vi "IO参数设置.vi"(8 "布尔文本.文本":string, 9 "section (optional)":string, 10 "监测项描述":string) -> (2 "增加？":bool, 3 "簇1输出":T1)   [LabVIEW 2016, in "环境动力监测库.lvlib"]
uses:
  <vilib>/Utility/miscctls.llb/LVPointTypeDef.ctl
  <vilib>/Utility/config.llb/NI_LVConfig.lvlib
panel:
  in  "声光告警启用":bool caption="声光告警"
  in  "参数配置":bool
  in  "采集设备":enum16{"PLC", "ZLAN", "ART"}(ring)
  in  "簇1输入":T1
  in  "返回":bool
  in  "增加":bool
  in  "告警参数":enum32{"禁用告警", "闭合告警", "断开告警"}(radio)
  in  "端口":T2(ring)
  in  "监测项描述":string
  # "基本设置"
  # "如:红外XX"
  # "传感器选择"
  # "端口选择"
  # "告警方式选择"
  # "声光告警选择"
  # "参数设置"
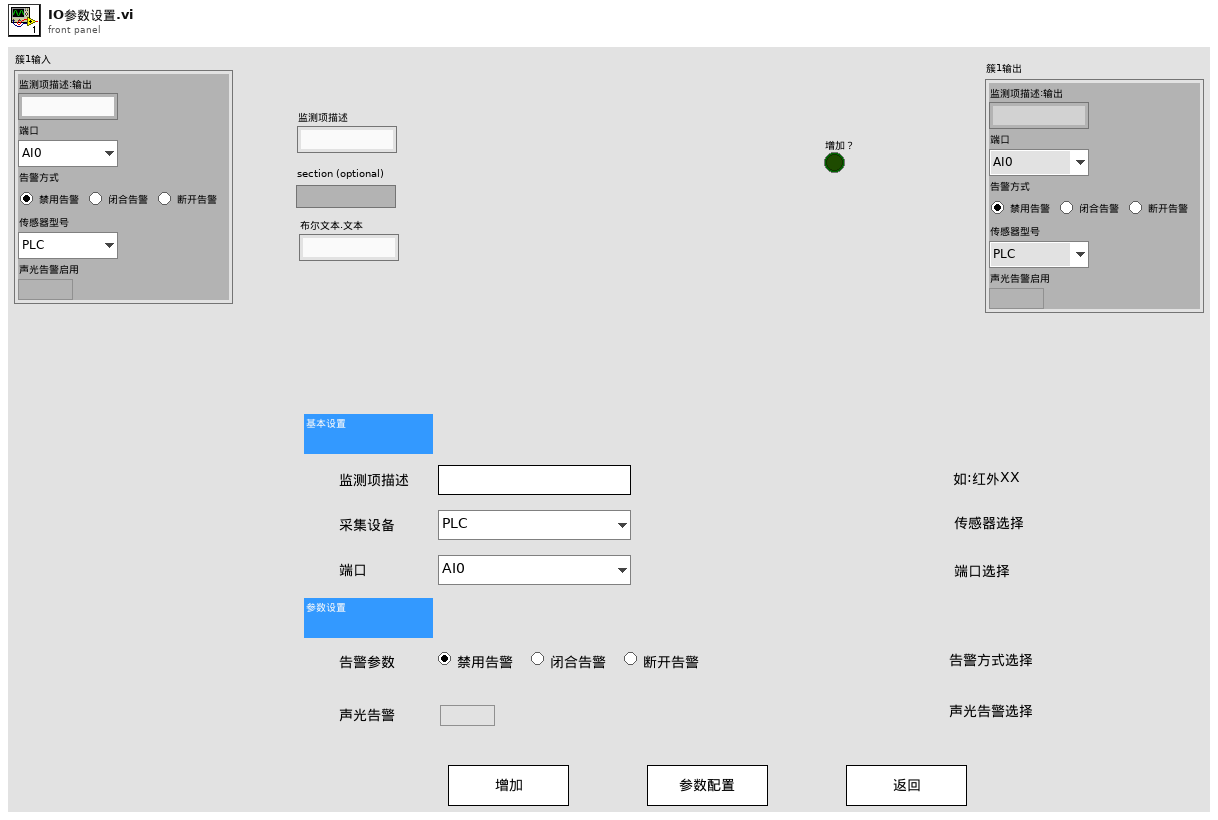
[diagram p1: front panel]
types:
  T1 = cluster{"监测项描述:输出":string, "端口":enum16{"AI0", "AI1", "AI2", "AI3", "AI4", "DI0", "DI1", "DI2", "DI3", "DI4", "DO0", "DO1", "DO2", "DO3", "DO4", "X0", "X1", "X2", "X3", "X4", "X5", "X6", "X7", "X8", "X9", "X10", "X11", "X12", "X13", "X14", "X15", "X16", "X17", "X18", "X19", "X20", "X21", "X22", "X23"}, "告警方式":enum32{"禁用告警", "闭合告警", "断开告警"}, "传感器型号":enum16{"PLC", "ZLAN", "ART"}, "声光告警启用":bool}
  T2 = enum16{"AI0", "AI1", "AI2", "AI3", "AI4", "DI0", "DI1", "DI2", "DI3", "DI4", "DO0", "DO1", "DO2", "DO3", "DO4", "X0", "X1", "X2", "X3", "X4", "X5", "X6", "X7", "X8", "X9", "X10", "X11", "X12", "X13", "X14", "X15", "X16", "X17", "X18", "X19", "X20", "X21", "X22", "X23"}
  T3 = cluster{"模板选择:":enum16{"定时简报", "无(不告警)", "通用声光告警", "通用语言告警", "通用短信告警", "通用电话告警", "通用邮件告警", "通用声光+语音+短信告警", "通用声光+短信+电话告警", "通用多方式告警", "通用全方式告警", "自动按类型", "非告警时段", "自定义"}, "预警保持时间\n(s):":i16, "重复告警时间\n(s):":i16, "告警发送方式:":cluster{"声光":bool, "语音":bool, "短信":bool, "彩信":bool, "电话":bool, "邮件":bool, "联动1":bool, "联动2":bool}, "告警时段选择:":enum16{"全时段告警", "工作日告警", "周六周日告警", "非告警时段", "自定义"}, "告警抓拍设置:":enum16{"无"}, "告警短信内容:":string, "告警电话内容:":string, "告警解除方式:":cluster{"声光":bool, "语音":bool, "短信":bool, "彩信":bool, "电话":bool, "邮件":bool, "联动1":bool, "联动2":bool}, "告警解除内容:":string, "信息接收人:":cluster{"管理员":bool, "普通用户":bool}}
  T4 = typedef "LVPointTypeDef.ctl" = cluster{"Horizontal":i16, "Vertical":i16}
  T5 = typedef "NI_LVConfig.lvlib/Config Data RefNum.ctl" = refnum<k1>
  T6 = enum8{"Enabled", "Disabled", "Disabled and Grayed Out"}
  T7 = cluster{"漏水监测配置":cluster{"监测项描述:输出":string, "端口:":enum16{"AI0", "AI1", "AI2", "AI3", "AI4", "DI0", "DI1", "DI2", "DI3", "DI4", "DO0", "DO1", "DO2", "DO3", "DO4", "X0", "X1", "X2", "X3", "X4", "X5", "X6", "X7", "X8", "X9", "X10", "X11", "X12", "X13", "X14", "X15", "X16", "X17", "X18", "X19", "X20", "X21", "X22", "X23"}, "告警参数:":enum32{"禁用告警", "闭合告警", "断开告警"}, "传感器型号:":enum16{"PLC", "ZLAN", "ART"}, "声光告警启用":bool}, "门禁开关监测配置":cluster{"监测项描述:输出":string, "端口:":enum16{"AI0", "AI1", "AI2", "AI3", "AI4", "DI0", "DI1", "DI2", "DI3", "DI4", "DO0", "DO1", "DO2", "DO3", "DO4", "X0", "X1", "X2", "X3", "X4", "X5", "X6", "X7", "X8", "X9", "X10", "X11", "X12", "X13", "X14", "X15", "X16", "X17", "X18", "X19", "X20", "X21", "X22", "X23"}, "告警参数:":enum32{"禁用告警", "闭合告警", "断开告警"}, "传感器型号:":enum16{"PLC", "ZLAN", "ART"}, "声光告警启用":bool}, "门禁开关监测配置2":cluster{"监测项描述:输出":string, "端口:":enum16{"AI0", "AI1", "AI2", "AI3", "AI4", "DI0", "DI1", "DI2", "DI3", "DI4", "DO0", "DO1", "DO2", "DO3", "DO4", "X0", "X1", "X2", "X3", "X4", "X5", "X6", "X7", "X8", "X9", "X10", "X11", "X12", "X13", "X14", "X15", "X16", "X17", "X18", "X19", "X20", "X21", "X22", "X23"}, "告警参数:":enum32{"禁用告警", "闭合告警", "断开告警"}, "传感器型号:":enum16{"PLC", "ZLAN", "ART"}, "声光告警启用":bool}, "温湿度监测配置":cluster{"监测项描述:输出":string, "端口:":enum16{"AI0", "AI1", "AI2", "AI3", "AI4", "DI0", "DI1", "DI2", "DI3", "DI4", "DO0", "DO1", "DO2", "DO3", "DO4", "X0", "X1", "X2", "X3", "X4", "X5", "X6", "X7", "X8", "X9", "X10", "X11", "X12", "X13", "X14", "X15", "X16", "X17", "X18", "X19", "X20", "X21", "X22", "X23"}, "告警参数:":enum32{"禁用告警", "闭合告警", "断开告警"}, "传感器型号:":enum16{"PLC", "ZLAN", "ART"}, "声光告警启用":bool}, "烟雾监测配置":cluster{"监测项描述:输出":string, "端口:":enum16{"AI0", "AI1", "AI2", "AI3", "AI4", "DI0", "DI1", "DI2", "DI3", "DI4", "DO0", "DO1", "DO2", "DO3", "DO4", "X0", "X1", "X2", "X3", "X4", "X5", "X6", "X7", "X8", "X9", "X10", "X11", "X12", "X13", "X14", "X15", "X16", "X17", "X18", "X19", "X20", "X21", "X22", "X23"}, "告警参数:":enum32{"禁用告警", "闭合告警", "断开告警"}, "传感器型号:":enum16{"PLC", "ZLAN", "ART"}, "声光告警启用":bool}, "冰箱监测配置":cluster{"监测项描述:输出":string, "端口:":enum16{"AI0", "AI1", "AI2", "AI3", "AI4", "DI0", "DI1", "DI2", "DI3", "DI4", "DO0", "DO1", "DO2", "DO3", "DO4", "X0", "X1", "X2", "X3", "X4", "X5", "X6", "X7", "X8", "X9", "X10", "X11", "X12", "X13", "X14", "X15", "X16", "X17", "X18", "X19", "X20", "X21", "X22", "X23"}, "告警参数:":enum32{"禁用告警", "闭合告警", "断开告警"}, "传感器型号:":enum16{"PLC", "ZLAN", "ART"}, "声光告警启用":bool}, "排气扇监测配置":cluster{"监测项描述:输出":string, "端口:":enum16{"AI0", "AI1", "AI2", "AI3", "AI4", "DI0", "DI1", "DI2", "DI3", "DI4", "DO0", "DO1", "DO2", "DO3", "DO4", "X0", "X1", "X2", "X3", "X4", "X5", "X6", "X7", "X8", "X9", "X10", "X11", "X12", "X13", "X14", "X15", "X16", "X17", "X18", "X19", "X20", "X21", "X22", "X23"}, "告警参数:":enum32{"禁用告警", "闭合告警", "断开告警"}, "传感器型号:":enum16{"PLC", "ZLAN", "ART"}, "声光告警启用":bool}, "红外入侵监测配置":cluster{"监测项描述:输出":string, "端口:":enum16{"AI0", "AI1", "AI2", "AI3", "AI4", "DI0", "DI1", "DI2", "DI3", "DI4", "DO0", "DO1", "DO2", "DO3", "DO4", "X0", "X1", "X2", "X3", "X4", "X5", "X6", "X7", "X8", "X9", "X10", "X11", "X12", "X13", "X14", "X15", "X16", "X17", "X18", "X19", "X20", "X21", "X22", "X23"}, "告警参数:":enum32{"禁用告警", "闭合告警", "断开告警"}, "传感器型号:":enum16{"PLC", "ZLAN", "ART"}, "声光告警启用":bool}, "振动监测配置":cluster{"监测项描述:输出":string, "端口:":enum16{"AI0", "AI1", "AI2", "AI3", "AI4", "DI0", "DI1", "DI2", "DI3", "DI4", "DO0", "DO1", "DO2", "DO3", "DO4", "X0", "X1", "X2", "X3", "X4", "X5", "X6", "X7", "X8", "X9", "X10", "X11", "X12", "X13", "X14", "X15", "X16", "X17", "X18", "X19", "X20", "X21", "X22", "X23"}, "告警参数:":enum32{"禁用告警", "闭合告警", "断开告警"}, "传感器型号:":enum16{"PLC", "ZLAN", "ART"}, "声光告警启用":bool}}
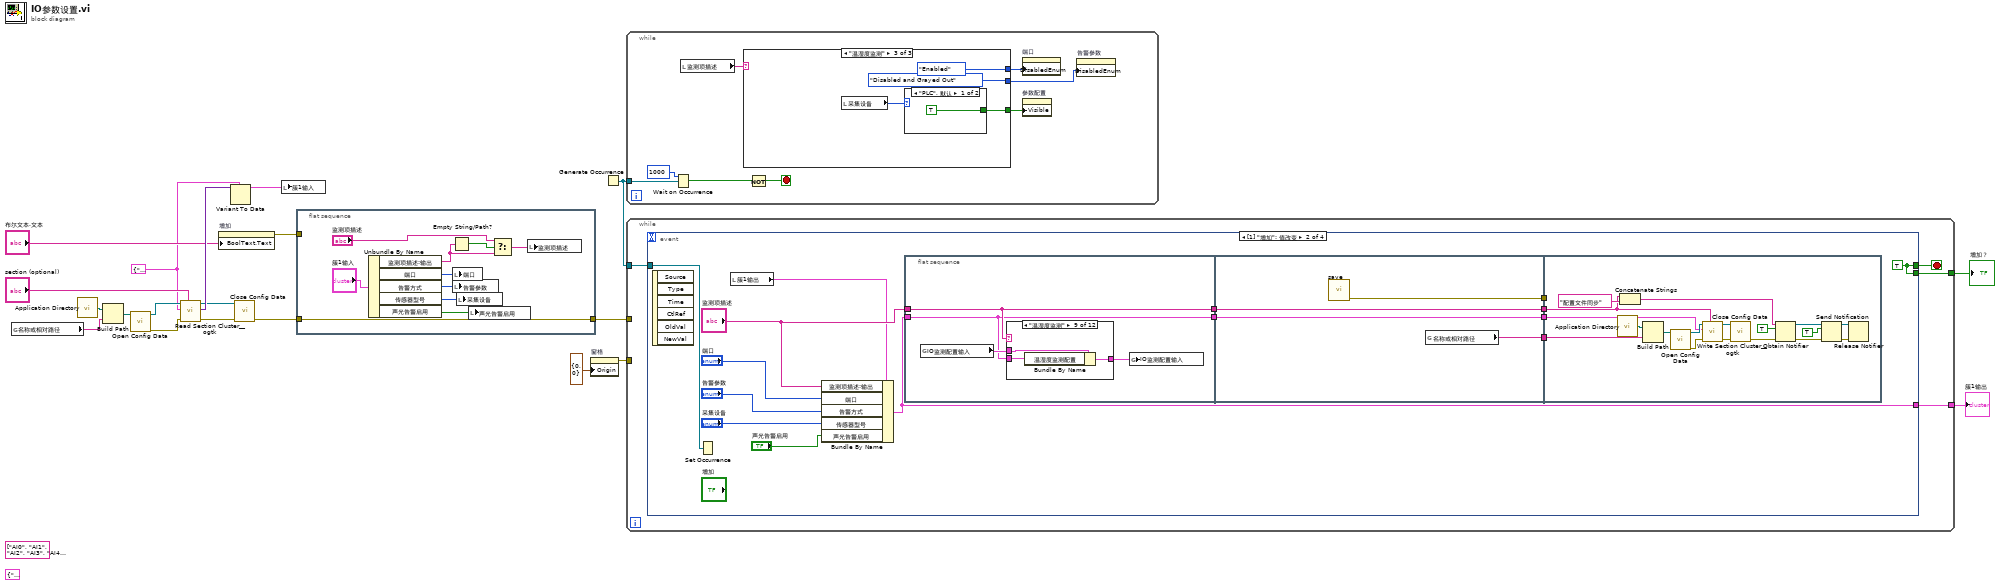
[diagram p0: block diagram]
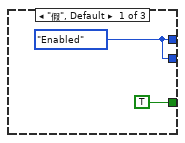
[diagram p2: hidden frame]
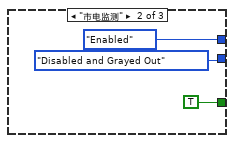
[diagram p3: hidden frame]
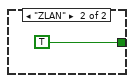
[diagram p4: hidden frame]
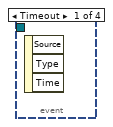
[diagram p5: hidden frame]
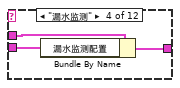
[diagram p9: hidden frame]
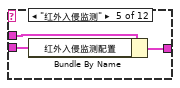
[diagram p10: hidden frame]
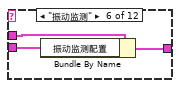
[diagram p11: hidden frame]
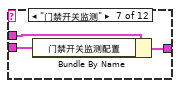
[diagram p12: hidden frame]
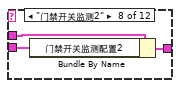
[diagram p13: hidden frame]
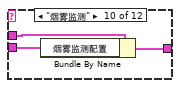
[diagram p14: hidden frame]
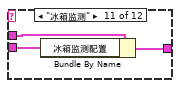
[diagram p15: hidden frame]
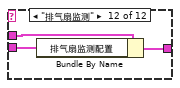
[diagram p16: hidden frame]
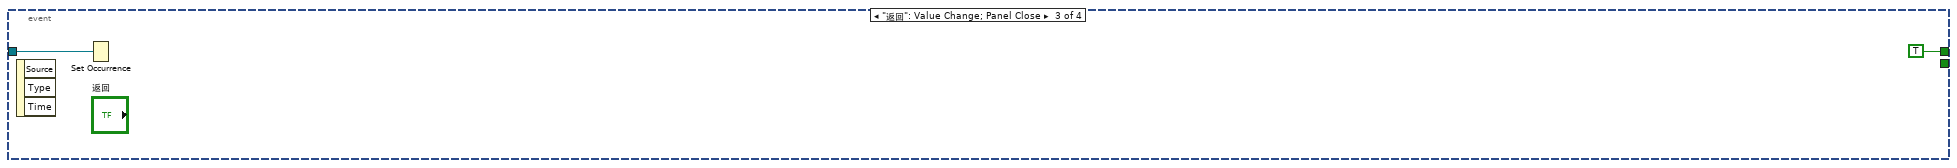
[diagram p17: hidden frame]
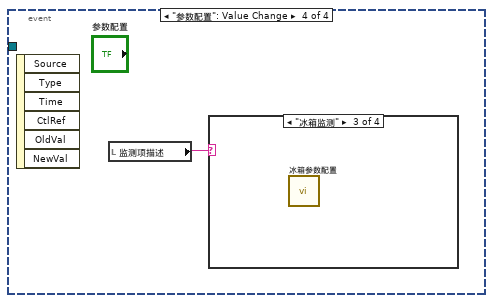
[diagram p18: hidden frame]
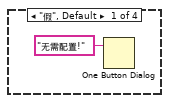
[diagram p19: hidden frame]
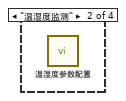
[diagram p20: hidden frame]
diagram:
  w2 = T1 {"监测项描述:输出"="", "端口"=enum."AI0", "告警方式"=enum."禁用告警", "传感器型号"=enum."PLC", "声光告警启用"=FALSE} ("簇1输入")
  (unwired) string[] ["AI0", "AI1", "AI2", "AI3", "AI4", "DI0", "DI1", "DI2", "DI3", "DI4", "DO0", "DO1", "DO2", "DO3", "DO4", "X0", "X1", "X2", "X3", "X4", "X5", "X6", "X7", "X8", "X9"] ("字符串[]")
  (unwired) T3 {"模板选择:"=enum."定时简报", "预警保持时间\n(s):"=0, "重复告警时间\n(s):"=0, "告警发送方式:"={"声光"=FALSE, "语音"=FALSE, "短信"=FALSE, "彩信"=FALSE, "电话"=FALSE, "邮件"=FALSE, "联动1"=FALSE, "联动2"=FALSE}, "告警时段选择:"=enum."全时段告警", "告警抓拍设置:"=enum."无", "告警短信内容:"="", "告警电话内容:"="", "告警解除方式:"={"声光"=FALSE, "语音"=FALSE, "短信"=FALSE, "彩信"=FALSE, "电话"=FALSE, "邮件"=FALSE, "联动1"=FALSE, "联动2"=FALSE}, "告警解除内容:"="", "信息接收人:"={"管理员"=FALSE, "普通用户"=FALSE}} ("数据")
  n1 = global read "内部交互全局变量.vi" "名称或相对路径"() -> (w1:string)
  n2 = call <vilib>:"Application Directory.vi"() -> ("Application Directory"=w14:path)
  n3 = Build Path(base path=w14, name or relative path=w1) -> (appended path=w15:path)
  n4 = call <vilib>:"Open Config Data.vi"("configuration file path"=w15) -> ("error out"=w16:errorcluster, "refnum"=w17:T5)  [unwired: 8 in, 1 out]
  n5 = call <userlib>:"Read Section Cluster__ogtk.vi"("section (optional)"="section (optional)", "error in (no error)"=w16, "Section Formatted Cluster Type"=w2, "refnum"=w17) -> ("error out"=w6:errorcluster, "Section Formatted Cluster"=w12:variant, "dup refnum"=w7:T5)  [unwired: 3 in, 2 out]
  n6 = property on="增加" class="Bool"("BoolText.Text"="布尔文本.文本") -> (error out=w8:errorcluster)  [unwired: 2 in, 1 out]
  n7 = Variant To Data(type=w2, Variant=w12) -> (data=w3:T1)  [unwired: 1 in, 1 out]
  n8 = call <vilib>:"Close Config Data.vi"("error in (no error)"=w6, "refnum"=w7) -> ("error out"=w11:errorcluster)  [unwired: 8 in, 1 out]
  n9 = local write "簇1输入"(w3) -> ()
  n10 = flat-sequence {
    tunnel: w11 -> [w29]
    tunnel: [w29] -> w10
    tunnel: w8 -> [_]
    frame #0 {
      n11 = Unbundle By Name("簇1输入") -> ("监测项描述:输出"=w26:string, "端口"=w24:T2, "告警方式"=w23:enum32{"禁用告警", "闭合告警", "断开告警"}, "传感器型号"=w22:enum16{"PLC", "ZLAN", "ART"}, "声光告警启用"=w21:bool)
      n12 = Empty String/Path?(string/path=w26) -> (empty?=w28:bool)
      n13 = local write "端口"(w24) -> ()
      n14 = local write "告警参数"(w23) -> ()
      n15 = local write "采集设备"(w22) -> ()
      n16 = local write "声光告警启用"(w21) -> ()
      n17 = Select(t="监测项描述", s=w28, f=w26) -> (s? t:f=w25:string)
      n18 = local write "监测项描述"(w25) -> ()
    }
  }
  n19 = property on="窗格" class="Pane"("Origin"=T4 {"Horizontal"=0, "Vertical"=0} ("原点")) -> (error out=w18:errorcluster)  [unwired: 2 in, 1 out]
  n20 = Generate Occurrence() -> (w5:refnum<k4>)
  n21 = while {
    tunnel: w5 -> [w36]
    stop <- w35 stop-if-true
    n22 = Wait on Occurrence(2:w36, 3:1000 ("毫秒超时(-1)")) -> (0:w37:bool)  [unwired: 1 in]
    n23 = local read "监测项描述"() -> (w34:string)
    n24 = case shown="\"温湿度监测\"" w34 {
      tunnel: [TRUE ("可见") TRUE ("可见") w46] -> w33
      tunnel: [w39 T6."Enabled" ("禁用") T6."Enabled" ("禁用")] -> w32
      tunnel: [w39 T6."Disabled and Grayed Out" ("禁用") T6."Disabled and Grayed Out" ("禁用")] -> w31
      frame "假", Default {
        w39 = T6."Enabled" ("禁用")
      }
      frame "市电监测" {
      }
      frame "温湿度监测" {
        n25 = local read "采集设备"() -> (w47:enum16{"PLC", "ZLAN", "ART"})
        n26 = case shown="\"PLC\", 默认" w47 {
          tunnel: [TRUE ("可见") TRUE ("可见")] -> w46
          frame "PLC", Default {
          }
          frame "ZLAN" {
          }
        }
      }
    }
    n27 = Not(x=w37) -> (.not. x?=w35:bool)
    n28 = property on="端口" class="Enum (严格)"("DisabledEnum"=w32) -> ()  [unwired: 2 in, 2 out]
    n29 = property on="参数配置" class="Bool"("Visible"=w33) -> ()  [unwired: 2 in, 2 out]
    n30 = property on="告警参数" class="RadioBtnsControl (严格)"("DisabledEnum"=w31) -> ()  [unwired: 2 in, 2 out]
  }
  n31 = while {
    tunnel: [w53] -> w4
    tunnel: [w51] -> w20
    tunnel: w18 -> [_]
    tunnel: w10 -> [_]
    tunnel: w5 -> [w50]
    stop <- w52 stop-if-true
    n32 = event shown="[1] \"增加\": 值改变" {
      selector: _ -> [_ _ _ _]
      dyn-events: _ -> [_ _ _ _]
      timeout: _ -> [_ _ _ _]
      tunnel: [_ w68 TRUE _] -> w52
      tunnel: [_ w61 _ _] -> w53
      tunnel: [_ w68 _ _] -> w51
      tunnel: w50 -> [_ w66 w125 _]
      event Timeout {
        n33 = event-data() -> ()  [unwired: 1 in, 3 out]
      }
      event "增加": Value Change {
        w68 = TRUE
        n34 = event-data() -> ()  [unwired: 1 in, 6 out]
        n35 = Set Occurrence(w66) -> ()
        n36 = local read "簇1输出"() -> (w65:T1)
        n37 = Bundle By Name(cluster=w65, "监测项描述:输出"="监测项描述", "端口"="端口", "告警方式"="告警参数", "传感器型号"="采集设备", "声光告警启用"="声光告警启用") -> (w61:T1)
        n38 = flat-sequence {
          tunnel: "监测项描述" -> [w70]
          tunnel: w61 -> [w69]
          tunnel: [w70] -> w60
          tunnel: [w69] -> w58
          tunnel: w60 -> [w106]
          tunnel: [w106] -> w59
          tunnel: w58 -> [w105]
          tunnel: [w105] -> w57
          tunnel: [w104] -> w55
          tunnel: [w103] -> w54
          tunnel: w59 -> [w109]
          tunnel: w57 -> [w111]
          tunnel: w55 -> [w107]
          tunnel: w54 -> [_]
          frame #0 {
            n39 = global read "断电保存全局变量.vi" "IO监测配置输入"() -> (w72:T7)
            n40 = case shown="\"温湿度监测\"" w70 {
              tunnel: w72 -> [w73 w74 w75 w78 w81 w84 w87 w90 w93 w96 w99 w102]
              tunnel: [w73 w74 w75 w77 w80 w83 w86 w89 w92 w95 w98 w101] -> w71
              tunnel: w69 -> [_ _ _ w76 w79 w82 w85 w88 w91 w94 w97 w100]
              frame "假", Default {
              }
              frame "市电监测" {
              }
              frame "空调监测" {
              }
              frame "漏水监测" {
                n41 = Bundle By Name(cluster=w78, "漏水监测配置"=w76) -> (w77:T7)
              }
              frame "红外入侵监测" {
                n42 = Bundle By Name(cluster=w81, "红外入侵监测配置"=w79) -> (w80:T7)
              }
              frame "振动监测" {
                n43 = Bundle By Name(cluster=w84, "振动监测配置"=w82) -> (w83:T7)
              }
              frame "门禁开关监测" {
                n44 = Bundle By Name(cluster=w87, "门禁开关监测配置"=w85) -> (w86:T7)
              }
              frame "门禁开关监测2" {
                n45 = Bundle By Name(cluster=w90, "门禁开关监测配置2"=w88) -> (w89:T7)
              }
              frame "温湿度监测" {
                n46 = Bundle By Name(cluster=w93, "温湿度监测配置"=w91) -> (w92:T7)
              }
              frame "烟雾监测" {
                n47 = Bundle By Name(cluster=w96, "烟雾监测配置"=w94) -> (w95:T7)
              }
              frame "冰箱监测" {
                n48 = Bundle By Name(cluster=w99, "冰箱监测配置"=w97) -> (w98:T7)
              }
              frame "排气扇监测" {
                n49 = Bundle By Name(cluster=w102, "排气扇监测配置"=w100) -> (w101:T7)
              }
            }
            n50 = global write "断电保存全局变量.vi" "IO监测配置输入"(w71) -> ()
          }
          frame #1 {
            n51 = call "save.vi"() -> ("error out"=w103:errorcluster)  [unwired: 11 in]
            n52 = global read "内部交互全局变量.vi" "名称或相对路径"() -> (w104:string)
          }
          frame #2 {
            n53 = call <vilib>:"Application Directory.vi"() -> ("Application Directory"=w114:path)
            n54 = Concatenate Strings(w109, "配置文件同步" ("名称（未命名）")) -> (w108:string)
            n55 = Build Path(base path=w114, name or relative path=w107) -> (appended path=w113:path)
            n56 = call <vilib>:"Open Config Data.vi"("configuration file path"=w113) -> ("error out"=w112:errorcluster, "refnum"=w124:T5)  [unwired: 8 in, 1 out]
            n57 = call <userlib>:"Write Section Cluster__ogtk.vi"("section (optional)"=w109, "error in (no error)"=w112, "Section Formatted Cluster"=w111, "refnum"=w124) -> ("error out"=w123:errorcluster, "dup refnum"=w122:T5)  [unwired: 6 in]
            n58 = call <vilib>:"Close Config Data.vi"("error in (no error)"=w123, "refnum"=w122) -> ("error out"=w119:errorcluster)  [unwired: 8 in, 1 out]
            n59 = Obtain Notifier(name (unnamed)=w108, notification data type=TRUE, error in (no error)=w119) -> (notifier out=w117:refnum<notifier>, error out=w118:errorcluster)  [unwired: 1 in, 1 out]
            n60 = Send Notification(notification=TRUE ("通知"), notifier=w117, error in (no error)=w118) -> (notifier out=w120:refnum<notifier>, error out=w121:errorcluster)
            n61 = Release Notifier(notifier=w120, error in (no error)=w121) -> ()  [unwired: 1 in, 3 out]
          }
        }
      }
      event "返回": Value Change; Panel Close {
        n62 = event-data() -> ()  [unwired: 1 in, 3 out]
        n63 = Set Occurrence(w125) -> ()
      }
      event "参数配置": Value Change {
        n64 = event-data() -> ()  [unwired: 1 in, 6 out]
        n65 = local read "监测项描述"() -> (w127:string)
        n66 = case shown="\"冰箱监测\"" w127 {
          frame "假", Default {
            n67 = One Button Dialog(message="无需配置!" ("消息")) -> ()  [unwired: 1 in, 1 out]
          }
          frame "温湿度监测" {
            n68 = call "温湿度参数配置.vi"() -> ()  [unwired: 12 in]
          }
          frame "冰箱监测" {
            n69 = call "冰箱参数配置.vi"() -> ()  [unwired: 12 in]
          }
          frame "排气扇监测" {
            n70 = call "排气扇参数配置.vi"() -> ()  [unwired: 12 in]
          }
        }
      }
    }
  }
  "增加？" <- w20
  "簇1输出" <- w4
